vi "Write Com Port.vi"(8 "error in (no error)":errorcluster, 10 "Com Port":refnum<visa-resource-name>, 11 "OsciloscopeClass in":refnum<class "OsciloscopeClass.lvclass">) -> (0 "error out":errorcluster, 3 "OsciloscopeClass out":refnum<class "OsciloscopeClass.lvclass">)   [LabVIEW 2020, in "OsciloscopeClass.lvclass"]
uses:
  OsciloscopeClass.lvclass
  OsciloscopeClass.lvclass/OsciloscopeClass.ctl
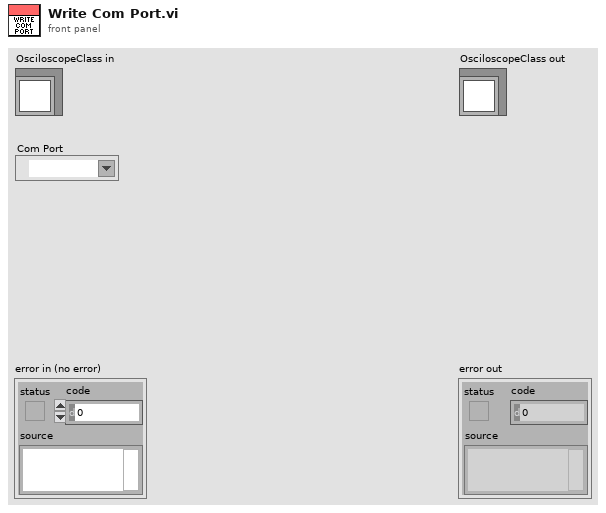
[diagram p1: front panel]
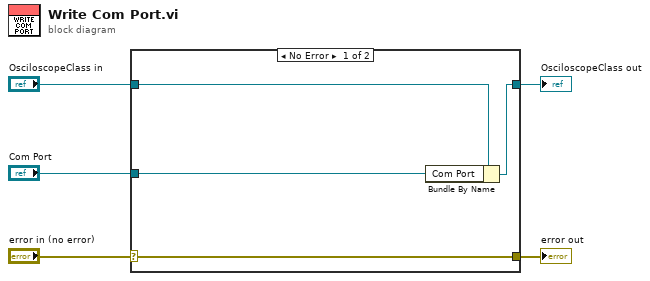
[diagram p0: block diagram]
diagram:
  n1 = case shown="No Error" "error in (no error)" {
    selector: "error in (no error)" -> [w9 w10]
    tunnel: [w9 w10] -> w4
    tunnel: [w7 w11] -> w2
    tunnel: "OsciloscopeClass in" -> [w8 w11]
    tunnel: "Com Port" -> [w6 _]
    frame No Error {
      n2 = Bundle By Name(cluster=w8, "Com Port"=w6) -> (w7:refnum<class "OsciloscopeClass.lvclass">)
    }
    frame Error {
    }
  }
  "error out" <- w4
  "OsciloscopeClass out" <- w2
